vi "AlliGator Format Slice Analysis Plots.vi"(9 "Plot Name Suffix":string, 11 "Result Plots Cluster":T1) -> (2 "Array of Plot Names":string[](array[string]), 3 "Array of Plots":cluster{"X Array":dbl[], "Y Array":dbl[]}[](array[cluster]), 5 "format string":string)   [LabVIEW 2021, in "AlliGator Lifetime & Other Parameters.lvlib"]
doc: "Gets a cluster of calculated plots and outputs them as an array, skipping empty plots (which haven't been calculated).\n\nThe associated names are also output, as well as a format string used to output a message listing these plots."
uses:
  Lifetime & Other Parameters/AlliGator Lifetime & Other Parameters.lvlib
  AlliGator Sliced Analysis Plots.ctl
  Graphs/XY Graph/XY Graph Plot Data.ctl
  Graphs/XY Graph/XY Graph Add-Ons.lvlib
  Strings/Strings.lvlib
  AlliGator Decay Fit Parameter Map.lvlib
panel:
  # "see the License on the block diagram (Ctrl+E or Window:Show Block Diagram)"
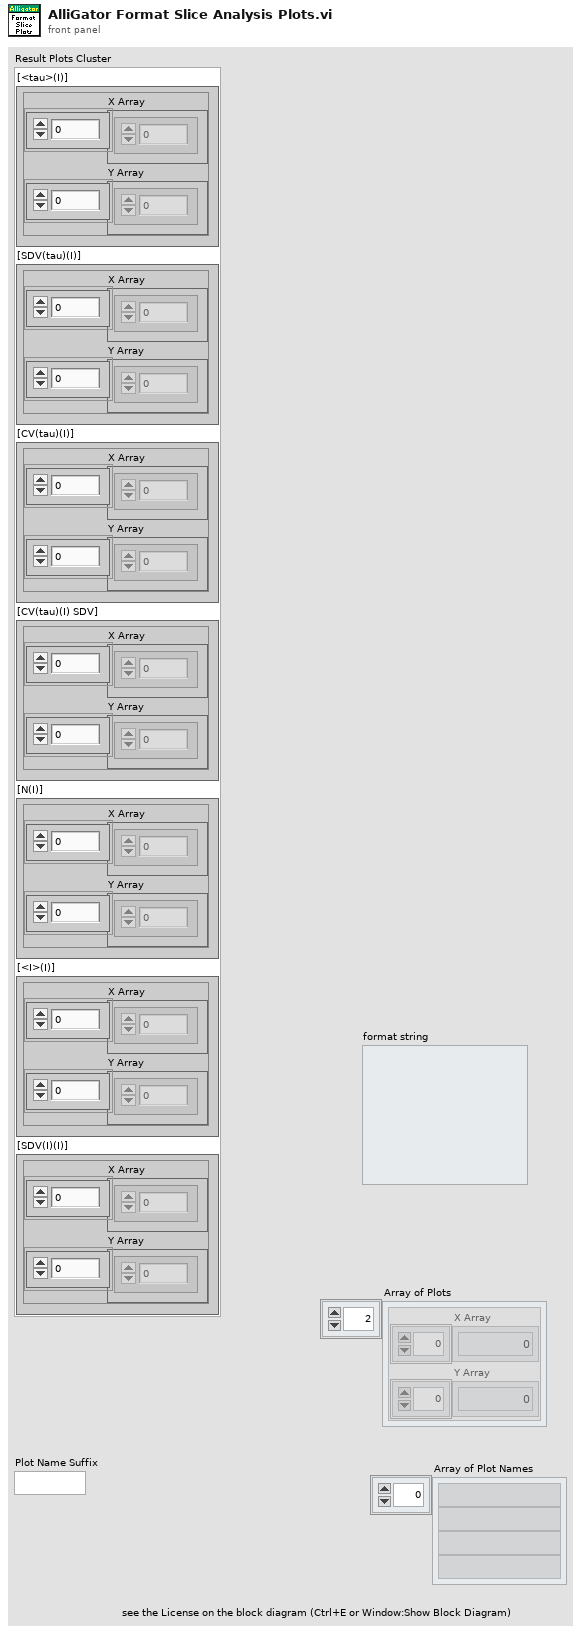
[diagram p1: front panel]
types:
  T1 = typedef "AlliGator Decay Fit Parameter Map.lvlib/AlliGator Sliced Analysis Plots.ctl" = cluster{"[<tau>(I)]":T2, "[SDV(tau)(I)]":T2, "[CV(tau)(I)]":T2, "[CV(tau)(I) SDV]":T2, "[N(I)]":T2, "[<I>(I)]":T2, "[SDV(I)(I)]":T2}
  T2 = typedef "XY Graph Add-Ons.lvlib/XY Graph Plot Data.ctl" = cluster{"X Array":dbl[], "Y Array":dbl[]}
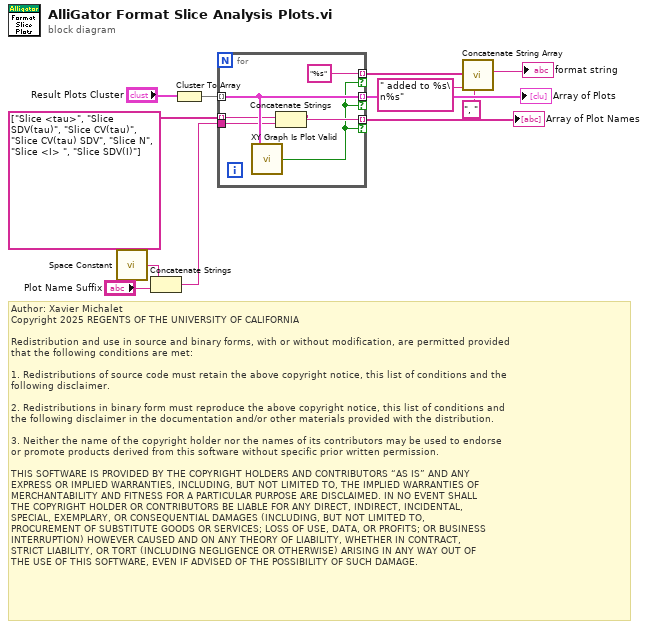
[diagram p0: block diagram]
diagram:
  # "Author: Xavier Michalet\nCopyright 2025 REGENTS OF THE UNIVERSITY OF CALIFORNIA\n\nRedistribution and use in source and binary forms, with or without modification, are permitted provided\nthat the following conditions are met:\n\n1. Redistributions of source code must retain the above copyright notice, this list of conditions and the\nfollowing disclaimer.\n\n2. Redistributions in binary form must reproduce the above copyright notice, this list of conditions and\nthe following disclaimer in the documentation and/or other materials provided with the distribution.\n\n3. Neither the name of the copyright holder nor the names of its contributors may be used to endorse \nor promote products derived from this software without specific prior written permission.\n\nTHIS SOFTWARE IS PROVIDED BY THE COPYRIGHT HOLDERS AND CONTRIBUTORS “AS IS” AND ANY \nEXPRESS OR IMPLIED WARRANTIES, INCLUDING, BUT NOT LIMITED TO, THE IMPLIED WARRANTIES OF\nMERCHANTABILITY AND FITNESS FOR A PARTICULAR PURPOSE ARE DISCLAIMED. IN NO EVENT SHALL\nTHE COPYRIGHT HOLDER OR CONTRIBUTORS BE LIABLE FOR ANY DIRECT, INDIRECT, INCIDENTAL, \nSPECIAL, EXEMPLARY, OR CONSEQUENTIAL DAMAGES (INCLUDING, BUT NOT LIMITED TO, \nPROCUREMENT OF SUBSTITUTE GOODS OR SERVICES; LOSS OF USE, DATA, OR PROFITS; OR BUSINESS\nINTERRUPTION) HOWEVER CAUSED AND ON ANY THEORY OF LIABILITY, WHETHER IN CONTRACT, \nSTRICT LIABILITY, OR TORT (INCLUDING NEGLIGENCE OR OTHERWISE) ARISING IN ANY WAY OUT OF\nTHE USE OF THIS SOFTWARE, EVEN IF ADVISED OF THE POSSIBILITY OF SUCH DAMAGE."
  n1 = call <vilib>:"Space Constant.vi"() -> ("String"=w6:string)
  n2 = Concatenate Strings(w6, "Plot Name Suffix") -> (w7:string)
  n3 = Cluster To Array(cluster="Result Plots Cluster") -> (array=w11:T2[])
  n4 = for {
    tunnel: w11 -> [w18] mode=indexing
    tunnel: string[] ["Slice <tau>", "Slice SDV(tau)", "Slice CV(tau)", "Slice CV(tau) SDV", "Slice N", "Slice <I> ", "Slice SDV(I)"] ("format string") -> [w17] mode=indexing
    tunnel: [w15] -> w1 mode=indexing if=w13
    tunnel: [w18] -> w9 mode=indexing if=w13
    tunnel: w7 -> [w16]
    tunnel: ["%s" ("format string")] -> w5 mode=indexing if=w13
    n5 = call "XY Graph Is Plot Valid.vi"("Plot"=w18) -> ("Is Valid Plot?"=w13:bool)  [unwired: 8 in]
    n6 = Concatenate Strings(w17, w16) -> (w15:string)
  }
  "Array of Plots" <- w9
  "Array of Plot Names" <- w1
  n7 = call "Concatenate String Array.vi"("Separator (TAB)"=", ", "Suffix (\"\")"=" added to %s\n%s" ("Suffix (\"\")"), "String Array"=w5) -> ("Formatted String"=→"format string":string)  [unwired: 8 in]
